vi "FormatChampHeader.vi"(9 "Caractère":string="=", 10 "NomChamp":string, 11 "Longueur":i32) -> (3 "String":string)   [LabVIEW 2020]
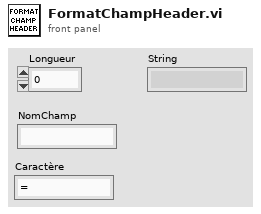
[diagram p1: front panel]
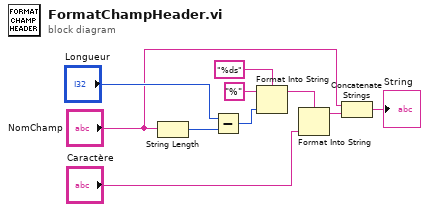
[diagram p0: block diagram]
diagram:
  n1 = String Length(string="NomChamp") -> (length=w1:i32)
  n2 = Subtract(x="Longueur", y=w1) -> (x-y=w4:i32)
  n3 = Format Into String(format string="%ds", initial string="%", w4) -> (resulting string=w5:string)  [unwired: 1 in, 1 out]
  n4 = Format Into String(format string=w5, "Caractère") -> (resulting string=w9:string)  [unwired: 2 in, 1 out]
  n5 = Concatenate Strings("NomChamp", w9) -> (→"String":string)
